vi "multichannel-capture.vi"() -> ()   [LabVIEW 2011]
uses:
  queue driver/Control.ctl
  queue driver/Control 2.ctl
  <vilib>/DAQmx/read.llb/DAQmx Read (Analog 2D DBL NChan NSamp).vi
  <vilib>/DAQmx/create/channels.llb/DAQmx Create Channel (AI-Voltage-Basic).vi
  <vilib>/DAQmx/configure/timing.llb/DAQmx Timing (Sample Clock).vi
  <vilib>/DAQmx/miscellaneous.llb/DAQmx Fill In Error Info.vi
  <vilib>/Utility/file.llb/Write To Spreadsheet File (DBL).vi
panel:
  out "INA current (V)":dbl
  out "discharge cur (V)":dbl
  out "Charge cur (V)":dbl
  in  "Output files Directory":path
  in  "physical channels":tag
  in  "exit":bool
  in  "capture":bool
  out "Waveform Chart":dbl[][](graph)
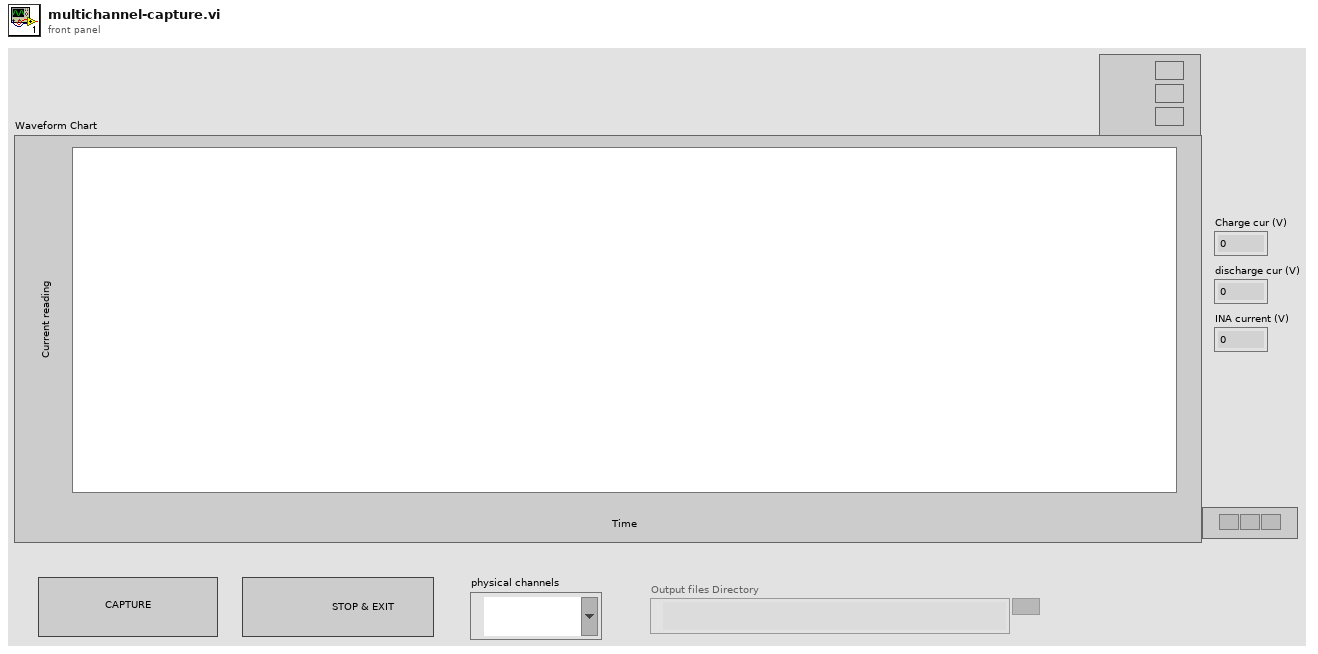
[diagram p1: front panel]
types:
  T1 = cluster{"device_task":refnum<k21>, "file_number":i32, "data":dbl[][], "file_directory":path, "file_name":string, "time_offset":dbl, "sample_rate":dbl, "capturing_data":bool, "incrementer\n":i32}
  T2 = typedef "Control 2.ctl" = enum16{"Initialize", "Poll", "Capture", "Store_to_file", "Exit"}
  T3 = typedef "Control.ctl" = enum16{"Create", "Enqueue-N", "Dequeue - 1 ", "Enstack - N", "Flush", "Release"}
  T4 = enum8{"Enabled", "Disabled", "Disabled and Grayed Out"}
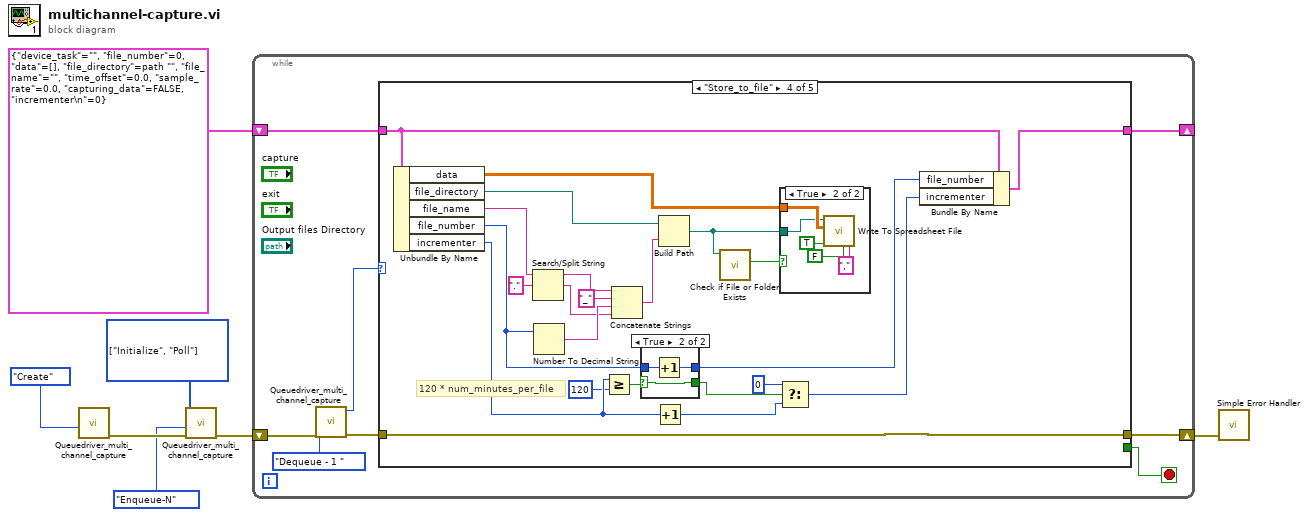
[diagram p0: block diagram]
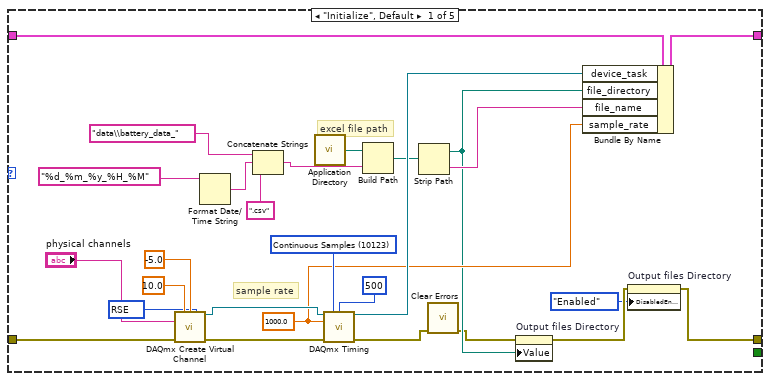
[diagram p2: hidden frame]
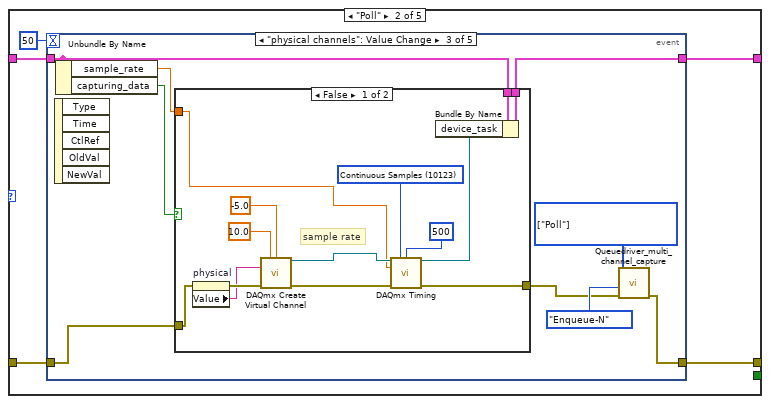
[diagram p3: hidden frame]
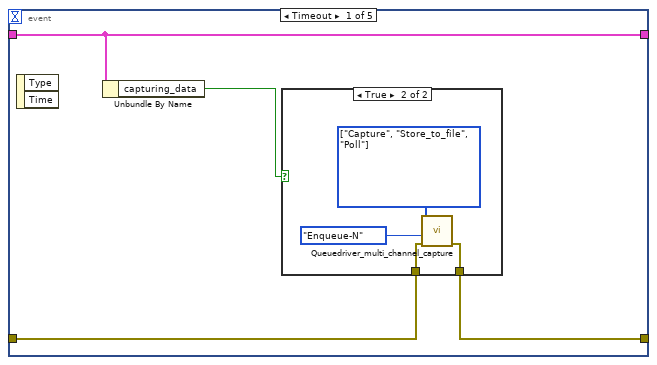
[diagram p4: hidden frame]
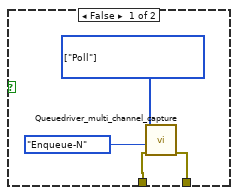
[diagram p5: hidden frame]
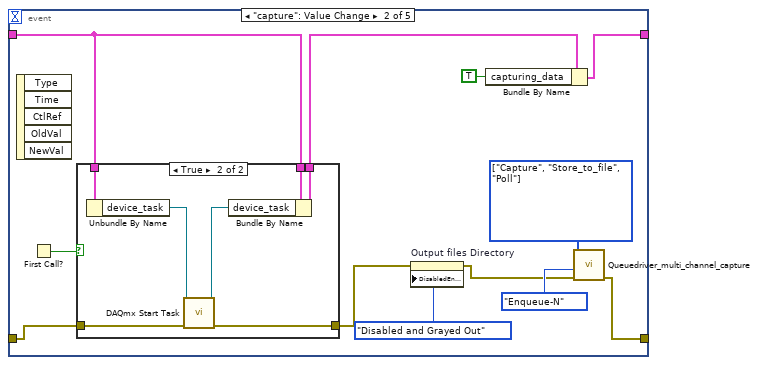
[diagram p6: hidden frame]
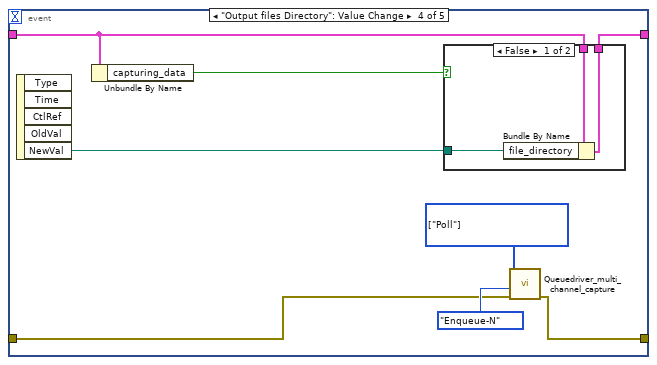
[diagram p9: hidden frame]
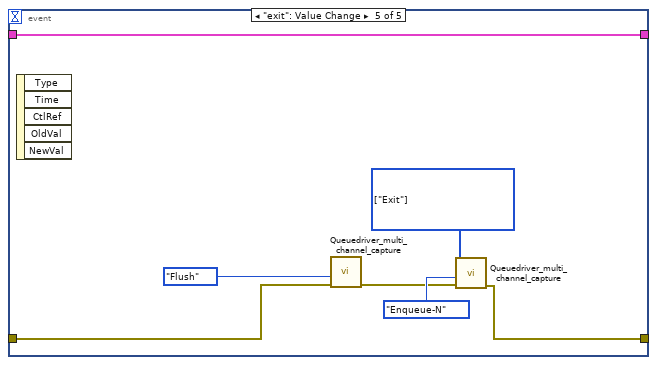
[diagram p11: hidden frame]
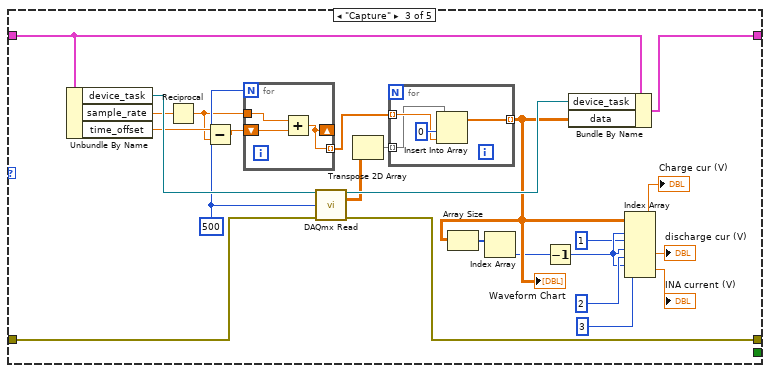
[diagram p12: hidden frame]
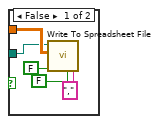
[diagram p13: hidden frame]
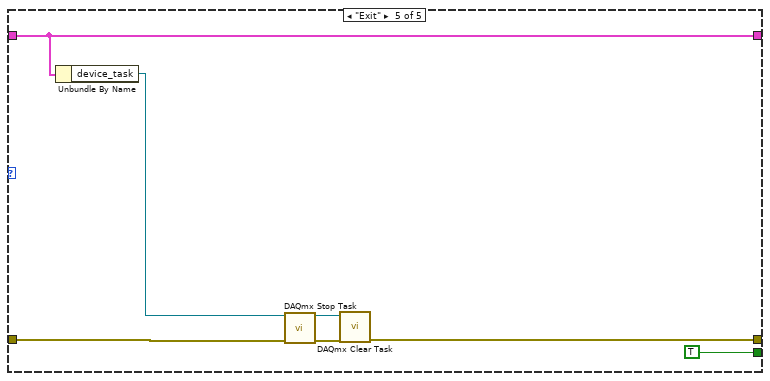
[diagram p15: hidden frame]
diagram:
  w4 = T2[] [enum."Initialize", enum."Poll"] items=["Initialize", "Poll", "Capture", "Store_to_file", "Exit"] ("Array")
  n1 = call "Queuedriver_multi_channel_capture.vi"("Operation"=Control."Create") -> ("error in 2"=w6:errorcluster)  [unwired: 9 in, 1 out]
  n2 = call "Queuedriver_multi_channel_capture.vi"("error in"=w6, "Operation"=Control."Enqueue-N", "Array"=w4) -> ("error in 2"=w3:errorcluster)  [unwired: 7 in, 1 out]
  n3 = while {
    shift-right: [w11] -> w2
    shift-left: w3 -> [w15]
    shift-right: [w9] -> _
    shift-left: T1 {"device_task"="", "file_number"=0, "data"=[], "file_directory"=path "", "file_name"="", "time_offset"=0.0, "sample_rate"=0.0, "capturing_data"=FALSE, "incrementer\n"=0} -> [w10]
    stop <- w8 stop-if-true
    n4 = call "Queuedriver_multi_channel_capture.vi"("error in"=w15, "Operation"=Control."Dequeue - 1 ") -> ("error in 2"=w12:errorcluster, "Enum"=w13:T2)  [unwired: 8 in]
    n5 = case shown="\"Store_to_file\"" w13 {
      tunnel: w12 -> [w39 w47 w148 w166 w197]
      tunnel: [w21 w46 w147 w166 w196] -> w11
      tunnel: w10 -> [w42 w45 w145 w168 w195]
      tunnel: [w41 w44 w144 w167 w195] -> w9
      tunnel: [_ _ _ _ TRUE] -> w8
      frame "Initialize", Default {
        w23 = 10083 items=["default"=-1, "RSE"=10083, "NRSE"=10078, "Differential"=10106, "Pseudodifferential"=12529] ("input terminal configuration")
        w33 = 10123 items=["Finite Samples"=10178, "Continuous Samples"=10123, "Hardware Timed Single Point"=12522] ("sample mode")
        w31 = 1000.0 ("rate")
        # "excel file path"
        # "sample rate"
        n6 = call-poly <vilib>:"DAQmx Create Virtual Channel.vi"("maximum value"=10.0, "minimum value"=-5.0 ("maximum value"), "input terminal configuration"=w23, "physical channels"="physical channels", "error in"=w39) -> ("task out"=w35:refnum<k21>, "error out"=w36:errorcluster)  [unwired: 9 in]
        n7 = Format Date/Time String(time format string (%c)="%d_%m_%y_%H_%M") -> (date/time string=w29:string)  [unwired: 2 in]
        n8 = Concatenate Strings("data\\battery_data_" ("name or relative path"), w29, ".csv" ("name or relative path")) -> (w30:string)
        n9 = call <vilib>:"Application Directory.vi"() -> ("Application Directory"=w18:path)
        n10 = call-poly <vilib>:"DAQmx Timing.vi"("task/channels in"=w35, "sample mode"=w33, "samples per channel"=500, "rate"=w31, "error in"=w36) -> ("task out"=w34:refnum<k21>, "error out"=w17:errorcluster)  [unwired: 9 in]
        n11 = Build Path(base path=w18, name or relative path=w30) -> (appended path=w25:path)
        n12 = Strip Path(path=w25) -> (stripped path=w19:path, name=w24:string)
        n13 = call <vilib>:"Clear Errors.vi"("error in (no error)"=w17) -> ("error out"=w16:errorcluster)  [unwired: 6 in]
        n14 = property on="Output files Directory" class="Path"(error in=w16, "Value"=w19) -> (error out=w22:errorcluster)  [unwired: 1 in, 1 out]
        n15 = Bundle By Name(cluster=w42, "device_task"=w34, "file_directory"=w19, "file_name"=w24, "sample_rate"=w31) -> (w41:T1)
        n16 = property on="Output files Directory" class="Path"(error in=w22, "DisabledEnum"=T4."Enabled" ("Disabled")) -> (error out=w21:errorcluster)  [unwired: 1 in, 1 out]
      }
      frame "Poll" {
        n17 = event shown="[2] \"physical channels\": Value Change" {
          selector: _ -> [_ _ _ _ _]
          dyn-events: _ -> [_ _ _ _ _]
          timeout: 50 -> [_ _ _ _ _]
          tunnel: w47 -> [w49 w67 w88 w108 w118]
          tunnel: [w48 w69 w82 w109 w121] -> w46
          tunnel: w45 -> [w51 w66 w87 w107 w124]
          tunnel: [w51 w64 w86 w113 w124] -> w44
          event Timeout {
            n18 = event-data() -> ()  [unwired: 1 in, 2 out]
            n19 = Unbundle By Name(w51) -> ("capturing_data"=w50:bool)
            n20 = case shown="True" w50 {
              tunnel: w49 -> [w53 w57]
              tunnel: [w52 w56] -> w48
              frame False {
                w55 = T2[] [enum."Poll"] items=["Initialize", "Poll", "Capture", "Store_to_file", "Exit"] ("Array")
                n21 = call "Queuedriver_multi_channel_capture.vi"("error in"=w53, "Operation"=Control."Enqueue-N", "Array"=w55) -> ("error in 2"=w52:errorcluster)  [unwired: 7 in, 1 out]
              }
              frame True {
                w59 = T2[] [enum."Capture", enum."Store_to_file", enum."Poll"] items=["Initialize", "Poll", "Capture", "Store_to_file", "Exit"] ("Array")
                n22 = call "Queuedriver_multi_channel_capture.vi"("error in"=w57, "Operation"=Control."Enqueue-N", "Array"=w59) -> ("error in 2"=w56:errorcluster)  [unwired: 7 in, 1 out]
              }
            }
          }
          event "capture": Value Change {
            w71 = T2[] [enum."Capture", enum."Store_to_file", enum."Poll"] items=["Initialize", "Poll", "Capture", "Store_to_file", "Exit"] ("Array")
            n23 = event-data() -> ()  [unwired: 1 in, 5 out]
            n24 = First Call?() -> (First Call?: T/F=w68:bool)
            n25 = case shown="True" w68 {
              tunnel: w66 -> [_ w80]
              tunnel: w67 -> [w72 w78]
              tunnel: [w72 w77] -> w62
              tunnel: w66 -> [w73 w76]
              tunnel: [w73 w75] -> w65
              frame False {
              }
              frame True {
                n26 = Unbundle By Name(w80) -> ("device_task"=w79:refnum<k21>)
                n27 = call <vilib>:"DAQmx Start Task.vi"("task/channels in"=w79, "error in"=w78) -> ("task out"=w74:refnum<k21>, "error out"=w77:errorcluster)  [unwired: 12 in]
                n28 = Bundle By Name(cluster=w76, "device_task"=w74) -> (w75:T1)
              }
            }
            n29 = property on="Output files Directory" class="Path"(error in=w62, "DisabledEnum"=T4."Disabled and Grayed Out" ("Disabled")) -> (error out=w61:errorcluster)  [unwired: 1 in, 1 out]
            n30 = Bundle By Name(cluster=w65, "capturing_data"=TRUE) -> (w64:T1)
            n31 = call "Queuedriver_multi_channel_capture.vi"("error in"=w61, "Operation"=Control."Enqueue-N", "Array"=w71) -> ("error in 2"=w69:errorcluster)  [unwired: 7 in, 1 out]
          }
          event "physical channels": Value Change {
            w85 = T2[] [enum."Poll"] items=["Initialize", "Poll", "Capture", "Store_to_file", "Exit"] ("Array")
            n32 = event-data() -> ()  [unwired: 1 in, 5 out]
            n33 = Unbundle By Name(w87) -> ("sample_rate"=w81:dbl, "capturing_data"=w89:bool)
            n34 = case shown="False" w89 {
              tunnel: w88 -> [w97 w105]
              tunnel: [w95 w105] -> w83
              tunnel: w87 -> [w94 w104]
              tunnel: [w93 w104] -> w86
              tunnel: w81 -> [w90 _]
              frame False {
                w99 = 10123 items=["Finite Samples"=10178, "Continuous Samples"=10123, "Hardware Timed Single Point"=12522] ("sample mode")
                # "sample rate"
                n35 = property on="physical" class="DAQmxName"(error in=w97) -> (error out=w96:errorcluster, "Value"=w91:string)  [unwired: 1 in, 1 out]
                n36 = call-poly <vilib>:"DAQmx Create Virtual Channel.vi"("maximum value"=10.0, "minimum value"=-5.0 ("maximum value"), "physical channels"=w91, "error in"=w96) -> ("task out"=w100:refnum<k21>, "error out"=w101:errorcluster)  [unwired: 10 in]
                n37 = call-poly <vilib>:"DAQmx Timing.vi"("task/channels in"=w100, "sample mode"=w99, "samples per channel"=500, "rate"=w90, "error in"=w101) -> ("task out"=w92:refnum<k21>, "error out"=w95:errorcluster)  [unwired: 9 in]
                n38 = Bundle By Name(cluster=w94, "device_task"=w92) -> (w93:T1)
              }
              frame True {
              }
            }
            n39 = call "Queuedriver_multi_channel_capture.vi"("error in"=w83, "Operation"=Control."Enqueue-N", "Array"=w85) -> ("error in 2"=w82:errorcluster)  [unwired: 7 in, 1 out]
          }
          event "Output files Directory": Value Change {
            w111 = T2[] [enum."Poll"] items=["Initialize", "Poll", "Capture", "Store_to_file", "Exit"] ("Array")
            n40 = event-data() -> ("NewVal"=w112:path)  [unwired: 1 in, 4 out]
            n41 = Unbundle By Name(w107) -> ("capturing_data"=w106:bool)
            n42 = case shown="False" w106 {
              tunnel: [w116 w117] -> w113
              tunnel: w112 -> [w115 _]
              tunnel: w107 -> [w114 w117]
              frame False {
                n43 = Bundle By Name(cluster=w114, "file_directory"=w115) -> (w116:T1)
              }
              frame True {
              }
            }
            n44 = call "Queuedriver_multi_channel_capture.vi"("error in"=w108, "Operation"=Control."Enqueue-N", "Array"=w111) -> ("error in 2"=w109:errorcluster)  [unwired: 7 in, 1 out]
          }
          event "exit": Value Change {
            w123 = T2[] [enum."Exit"] items=["Initialize", "Poll", "Capture", "Store_to_file", "Exit"] ("Array")
            n45 = event-data() -> ()  [unwired: 1 in, 5 out]
            n46 = call "Queuedriver_multi_channel_capture.vi"("error in"=w118, "Operation"=Control."Flush") -> ("error in 2"=w120:errorcluster)  [unwired: 8 in, 1 out]
            n47 = call "Queuedriver_multi_channel_capture.vi"("error in"=w120, "Operation"=Control."Enqueue-N", "Array"=w123) -> ("error in 2"=w121:errorcluster)  [unwired: 7 in, 1 out]
          }
        }
      }
      frame "Capture" {
        w141 = 500 ("number of samples per channel")
        n48 = Unbundle By Name(w145) -> ("device_task"=w146:refnum<k21>, "sample_rate"=w142:dbl, "time_offset"=w140:dbl)
        n49 = Reciprocal(x=w142) -> (1/x=w139:dbl)
        n50 = Subtract(x=w140, y=w139) -> (x-y=w138:dbl)
        n51 = for {
          N: w141 -> [_]
          tunnel: w139 -> [w154]
          shift-right: [w153] -> _
          shift-left: w138 -> [w155]
          tunnel: [w153] -> w137 mode=indexing
          n52 = Add(x=w154, y=w155) -> (x+y=w153:dbl)
        }
        n53 = call-poly <vilib>:"DAQmx Read.vi"("task/channels in"=w146, "number of samples per channel"=w141, "error in"=w148) -> ("task out"=w143:refnum<k21>, "data"=w135:dbl[][], "error out"=w147:errorcluster)  [unwired: 10 in]
        n54 = Transpose 2D Array(2D array=w135) -> (transposed array=w136:dbl[][])
        n55 = for {
          tunnel: w137 -> [w151] mode=indexing
          tunnel: w136 -> [w150] mode=indexing
          tunnel: [w149] -> w134 mode=indexing
          n56 = Insert Into Array(array=w150, index=0, new element=w151) -> (w149:dbl[])
        }
        "Waveform Chart" <- w134
        n57 = Array Size(array=w134) -> (size(s)=w133:i32[])
        n58 = Index Array(array=w133) -> (element=w128:i32)  [unwired: 1 in]
        n59 = Decrement(x=w128) -> (x-1=w127:i32)
        n60 = Bundle By Name(cluster=w145, "device_task"=w143, "data"=w134) -> (w144:T1)
        n61 = Index Array(array=w134, index (row) #1=w127, index (col) #1=1 ("disabled index (col)"), index (row) #2=w127, index (col) #2=2 ("disabled index (col)"), index (row) #3=w127, index (col) #3=3 ("disabled index (col)")) -> (element #1=→"Charge cur (V)":dbl, element #2=→"discharge cur (V)":dbl, element #3=→"INA current (V)":dbl)
      }
      frame "Store_to_file" {
        # "120 * num_minutes_per_file"
        n62 = Unbundle By Name(w168) -> ("data"=w178:dbl[][], "file_directory"=w177:path, "file_name"=w176:string, "file_number"=w169:i32, "incrementer"=w163:i32)
        n63 = Search/Split String(string=w176, search string/char (-)=".") -> (substring before match=w174:string, match + rest of string=w171:string)  [unwired: 1 in, 1 out]
        n64 = Number To Decimal String(number=w169) -> (decimal integer string=w172:string)  [unwired: 1 in]
        n65 = Greater Or Equal?(x=w163, y=120) -> (x >= y?=w164:bool)
        n66 = Concatenate Strings(w174, "_" ("string"), w172, w171) -> (w170:string)
        n67 = case shown="True" w164 {
          selector: w164 -> [w189 w191]
          tunnel: w169 -> [w190 w193]
          tunnel: [w190 w192] -> w165
          tunnel: [w189 w191] -> w161
          frame False {
          }
          frame True {
            n68 = Increment(x=w193) -> (x+1=w192:i32)
          }
        }
        n69 = Increment(x=w163) -> (x+1=w160:i32)
        n70 = Build Path(base path=w177, name or relative path=w170) -> (appended path=w157:path)
        n71 = call <vilib>:"Check if File or Folder Exists.vi"("path"=w157) -> ("file or folder exists?"=w156:bool)  [unwired: 8 in, 2 out]
        n72 = case shown="True" w156 {
          tunnel: w178 -> [w180 w188]
          tunnel: w157 -> [w179 w184]
          frame False {
            n73 = call-poly <vilib>:"Write To Spreadsheet File.vi"("delimiter (\\t)"="," ("delimiter (\\t)"), "transpose? (no:F)"=FALSE, "append to file? (new file:F)"=FALSE, "2D data"=w180, "file path (dialog if empty)"=w179) -> ()  [unwired: 3 in, 1 out]
          }
          frame True {
            n74 = call-poly <vilib>:"Write To Spreadsheet File.vi"("delimiter (\\t)"="," ("delimiter (\\t)"), "transpose? (no:F)"=FALSE, "append to file? (new file:F)"=TRUE, "2D data"=w188, "file path (dialog if empty)"=w184) -> ()  [unwired: 3 in, 1 out]
          }
        }
        n75 = Select(t=0, s=w161, f=w160) -> (s? t:f=w159:i32)
        n76 = Bundle By Name(cluster=w168, "file_number"=w165, "incrementer"=w159) -> (w167:T1)
      }
      frame "Exit" {
        n77 = Unbundle By Name(w195) -> ("device_task"=w194:refnum<k21>)
        n78 = call <vilib>:"DAQmx Stop Task.vi"("task/channels in"=w194, "error in"=w197) -> ("task out"=w198:refnum<k21>, "error out"=w199:errorcluster)  [unwired: 12 in]
        n79 = call <vilib>:"DAQmx Clear Task.vi"("task in"=w198, "error in"=w199) -> ("error out"=w196:errorcluster)  [unwired: 13 in]
      }
    }
  }
  n80 = call <vilib>:"Simple Error Handler.vi"("error in (no error)"=w2) -> ()  [unwired: 4 in, 5 out]
